vi "ARXOLAB LABVIEW 2018.vi"() -> ()   [LabVIEW 2017]
uses:
  <vilib>/Instr/_visa.llb/VISA Configure Serial Port (Instr).vi
panel:
  out "?":string
  out "?":string
  out "?":dbl
  out "?":dbl
  out "Presion Atmosferica":dbl(knob) scale=0.0..3000.0
  out "Altura Aproximada":dbl(slide) scale=0.0..6060.0
  out "?":dbl
  out "?":dbl
  out "?":dbl
  in  "?":bool
  out "Temperatura Analoga":dbl(slide) scale=0.0..50.0
  out "Temperatura Digital":dbl(slide) scale=0.0..50.0
  out "Húmedad":dbl(knob) scale=0.0..100.0
  in  "?":refnum<visa-resource-name>
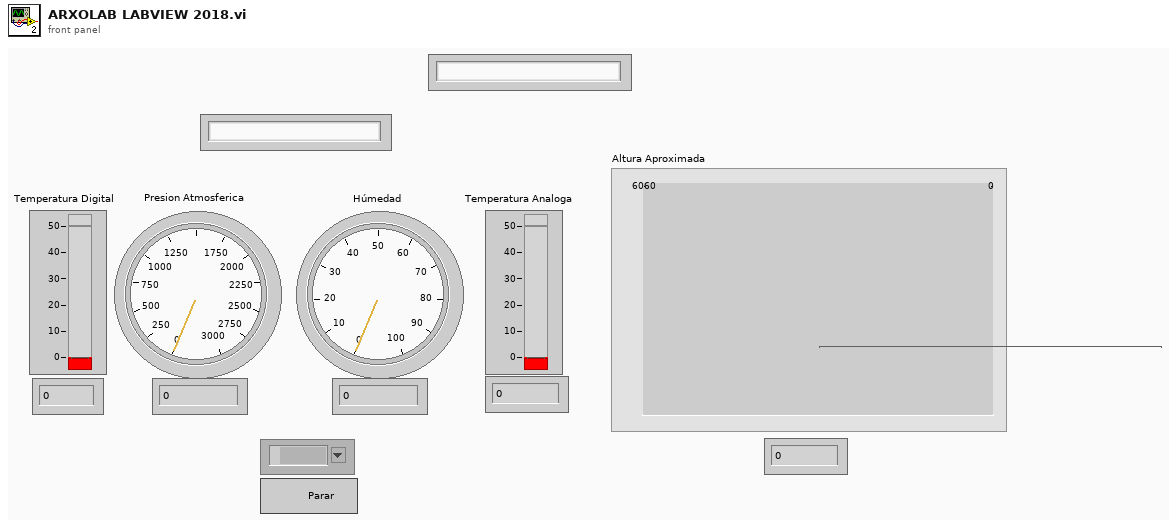
[diagram p1: front panel]
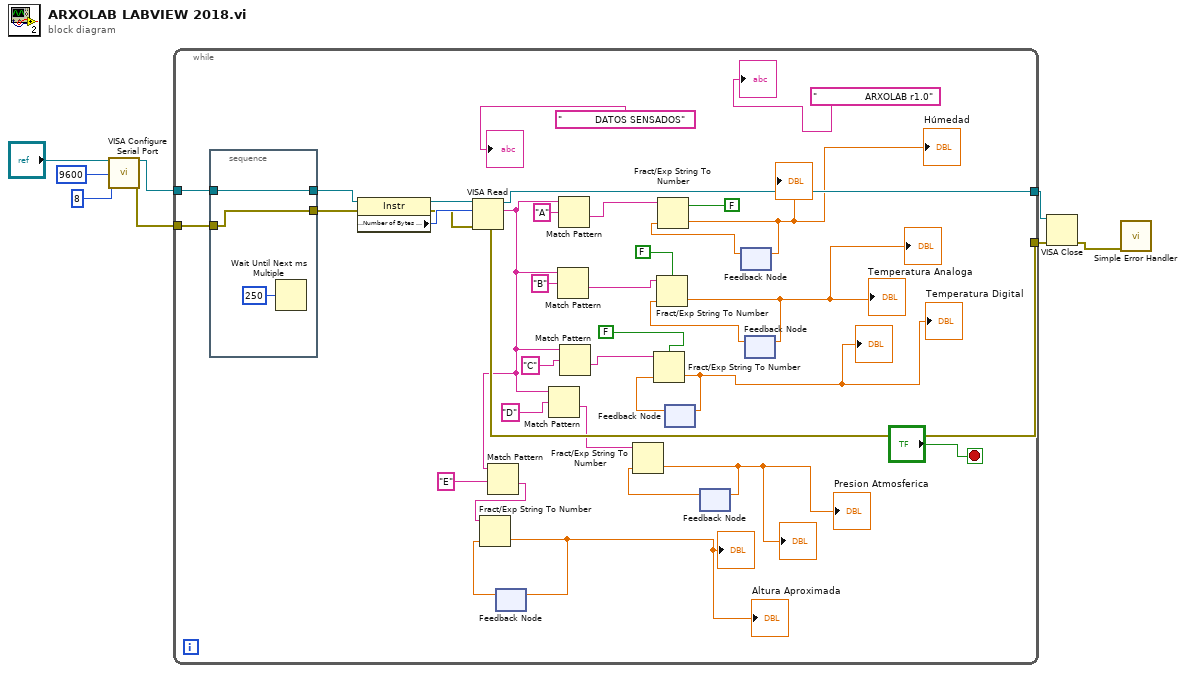
[diagram p0: block diagram]
diagram:
  n1 = call-poly "VISA Configure Serial Port"("VISA resource name"="?", "baud rate (9600)"=u32 9600, "data bits (8)"=u16 8) -> ("VISA resource name out"=w5:refnum<visa-resource-name>, "error out"=w4:errorcluster)  [unwired: 11 in]
  n2 = while {
    tunnel: w5 -> [w44]
    tunnel: w4 -> [w42]
    tunnel: [w29] -> w3
    tunnel: [w28] -> w2
    stop <- "?" stop-if-true
    n3 = stacked-sequence {
      tunnel: w44 -> [w47]
      tunnel: [w47] -> w43
      tunnel: w42 -> [w46]
      tunnel: [w46] -> w41
      frame #0 {
        n4 = Wait Until Next ms Multiple(millisecond multiple=u32 250) -> ()  [unwired: 1 out]
      }
    }
    n5 = property class="Instr"(reference=w43, error in=w41) -> (reference out=w40:refnum<visa-resource-name>, error out=w38:errorcluster, "Serial Settings:Number of Bytes at Serial Port"=w39:u32)
    n6 = VISA Read(VISA resource name=w40, byte count=w39, error in (no error)=w38) -> (VISA resource name out=w29:refnum<visa-resource-name>, read buffer=w14:string, error out=w28:errorcluster)  [unwired: 1 out]
    n7 = Match Pattern(string=w14, regular expression="E") -> (after substring=w13:string)  [unwired: 1 in, 3 out]
    n8 = feedback #1() -> (w12:dbl)  [unwired: 1 in]
    n9 = Fract/Exp String To Number(string=w13, default (0 dbl)=w12) -> (number=w10:dbl)  [unwired: 2 in, 1 out]
    "Altura Aproximada" <- w10
    "?" <- w10
    n10 = feedback-in #1(w10) -> ()
    n11 = Match Pattern(string=w14, regular expression="D") -> (after substring=w18:string)  [unwired: 1 in, 3 out]
    n12 = Match Pattern(string=w14, regular expression="B") -> (after substring=w34:string)  [unwired: 1 in, 3 out]
    n13 = Match Pattern(string=w14, regular expression="A") -> (after substring=w35:string)  [unwired: 1 in, 3 out]
    n14 = Match Pattern(string=w14, regular expression="C") -> (after substring=w26:string)  [unwired: 1 in, 3 out]
    n15 = feedback #2() -> (w25:dbl)  [unwired: 1 in]
    n16 = Fract/Exp String To Number(use system decimal point (T)=FALSE, string=w26, default (0 dbl)=w25) -> (number=w20:dbl)  [unwired: 1 in, 1 out]
    "Temperatura Digital" <- w20
    "?" <- w20
    n17 = feedback-in #2(w20) -> ()
    n18 = feedback #3() -> (w17:dbl)  [unwired: 1 in]
    n19 = Fract/Exp String To Number(string=w18, default (0 dbl)=w17) -> (number=w16:dbl)  [unwired: 2 in, 1 out]
    "?" <- w16
    "Presion Atmosferica" <- w16
    n20 = feedback-in #3(w16) -> ()
    n21 = feedback #4() -> (w31:dbl)  [unwired: 1 in]
    n22 = Fract/Exp String To Number(use system decimal point (T)=FALSE, string=w35, default (0 dbl)=w31) -> (number=w22:dbl)  [unwired: 1 in, 1 out]
    "Húmedad" <- w22
    "?" <- w22
    n23 = feedback-in #4(w22) -> ()
    n24 = feedback #5() -> (w30:dbl)  [unwired: 1 in]
    n25 = Fract/Exp String To Number(use system decimal point (T)=FALSE, string=w34, default (0 dbl)=w30) -> (number=w21:dbl)  [unwired: 1 in, 1 out]
    "Temperatura Analoga" <- w21
    "?" <- w21
    n26 = feedback-in #5(w21) -> ()
    "?" <- "           DATOS SENSADOS"
    "?" <- "                ARXOLAB r1.0"
  }
  n27 = VISA Close(VISA resource name=w3, error in (no error)=w2) -> (error out=w1:errorcluster)
  n28 = call <vilib>:"Simple Error Handler.vi"("error in (no error)"=w1) -> ()  [unwired: 4 in, 5 out]
